vi "1.2.2-ReadSerial.vi"() -> ()   [LabVIEW 2010]
uses:
  2-Low Neurons/2.2-Where Sensor Typedef.ctl
  <vilib>/eio/EIOMethodNode/EIOMethodNode.xnode
  <vilib>/rvi/eio/nirviEIOMethodImplementation/nirviEIOMethodImplementation.xnode
  <vilib>/rvi/eio/common/nirviEmuClasses.ctl
  1.0-Hindbrain Global.vi
  <vilib>/rvi/eio/common/nirviEmuTemplateMethod_noerrors.vi
panel:
  in  "ASCII: Command type":u8[](array[numeric])=[86, 78, 82, 82, 79, 44]
  out "Yaw":i16
  out "RAW Data":u8
  # "VNRRG,: 86 - 78 - 82 - 82 - 71 - 44"
  # "VNYPR,: 86 - 78 - 89 - 80 - 82 - 44"
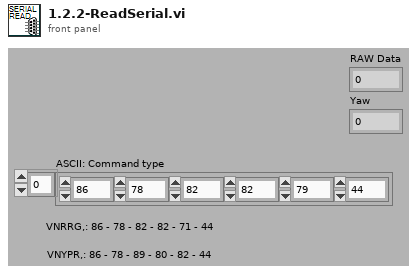
[diagram p1: front panel]
types:
  T1 = typedef "2.2-Where Sensor Typedef.ctl" = cluster{"INS X":i16, "INS Y":i16, "INS Z":i16, "INS Yaw":i16, "INS Raw":i8}
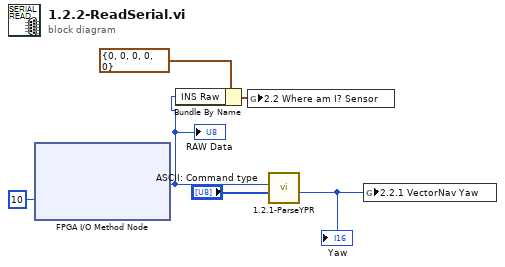
[diagram p0: block diagram]
diagram:
  n1 = xnode "FPGA I/O Method Node"("Timeout (ms)"=10) -> ("Data"=w6:u8)  [unwired: 1 in, 2 out]
  "RAW Data" <- w6
  n2 = Bundle By Name(cluster=T1 {"INS X"=0, "INS Y"=0, "INS Z"=0, "INS Yaw"=0, "INS Raw"=0} ("2.2 Where am I? Sensor"), "INS Raw"=w6) -> (w5:T1)
  n3 = global write "1.0-Hindbrain Global.vi" "2.2 Where am I? Sensor"(w5) -> ()
  n4 = call "1.2.1-ParseYPR.vi"("ASCII: VNYPR,"="ASCII: Command type", "Serial Byte"=w6) -> ("Yaw"=w2:i16)  [unwired: 9 in]
  "Yaw" <- w2
  n5 = global write "1.0-Hindbrain Global.vi" "2.2.1 VectorNav Yaw"(w2) -> ()
